vi "test Find Missing Hardware Modules.vi"(8 "error in (no error)":errorcluster, 11 "TestCase in":refnum<class "Routing and Faulting Validation Unit Tests.lvclass">) -> (0 "error out":errorcluster, 3 "TestCase out":refnum<class "Routing and Faulting Validation Unit Tests.lvclass">)   [LabVIEW 2020, in "Routing and Faulting Validation Unit Tests.lvclass"]
uses:
  Routing and Faulting Validation Unit Tests.lvclass
  Routing and Faulting Validation Unit Tests.lvclass/Routing and Faulting Validation Unit Tests.ctl
  <vilib>/addons/_JKI Toolkits/VI Tester/TestCase.llb/TestCase.lvclass
  Routing and Faulting Scripting.lvlib
  C:/Program Files (x86)/National Instruments/LabVIEW 2020/vi.lib/addons/_JKI Toolkits/VI Tester/TestCase.llb/TestCase.lvclass
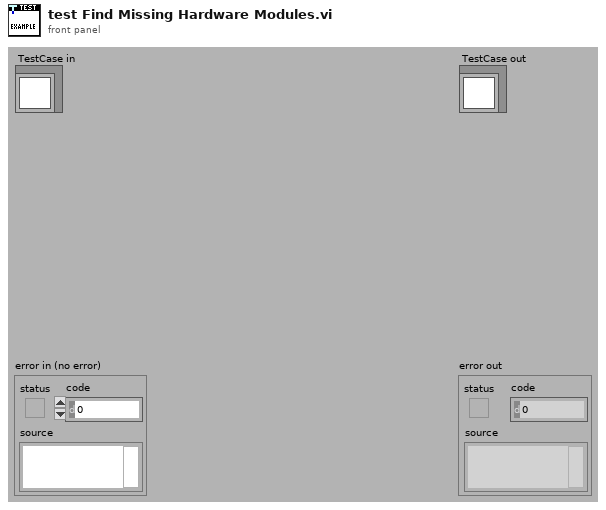
[diagram p1: front panel]
types:
  T1 = typedef "Custom Device API.lvlib/Custom Device Item Ref.ctl" = u64
  T2 = typedef "Routing and Faulting Scripting.lvlib/Validation Information.ctl" = cluster{"Missing Modules":variant, "Module Connection Map":variant, "Unused Modules":variant}
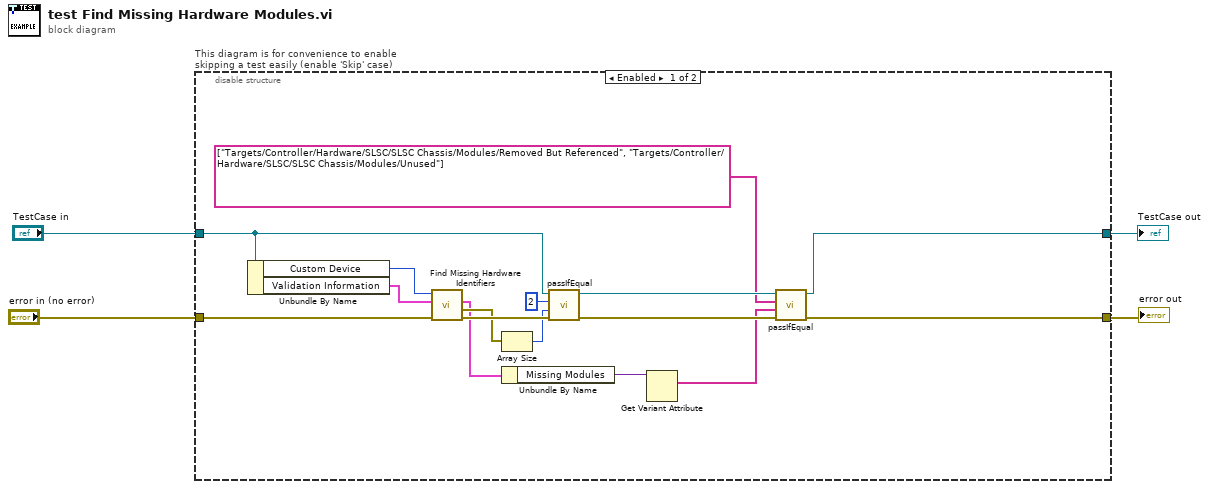
[diagram p0: block diagram]
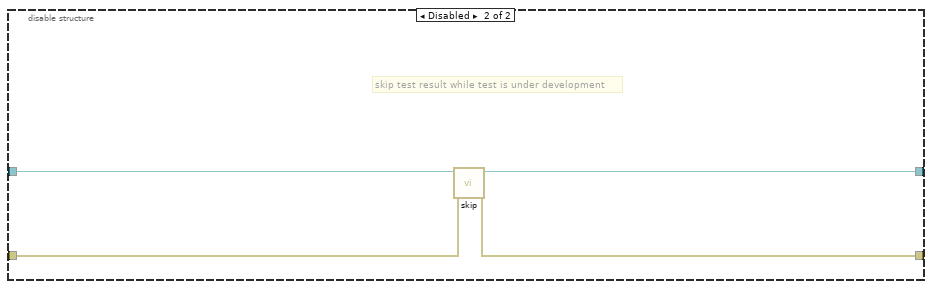
[diagram p2: hidden frame]
diagram:
  n1 = disable-structure "This diagram is for convenience to enable skipping a test easily (enable 'Skip' case)" shown="Enabled" {
    disable-tunnel: "TestCase in" -> [w13 w24]
    disable-tunnel: [w8 w22] -> w1
    disable-tunnel: [w7 w23] -> w3
    disable-tunnel: "error in (no error)" -> [w20 w21]
    frame Enabled {
      n2 = Unbundle By Name(w13) -> ("Custom Device"=w19:T1, "Validation Information"=w18:T2)
      n3 = call "Find Missing Hardware Identifiers.vi"("error in"=w20, "validation information in"=w18, "routing and faulting in"=w19) -> ("error out"=w17:errorcluster, "identifier errors"=w16:errorcluster[], "validation information out"=w12:T2)  [unwired: 5 in, 1 out]
      n4 = Array Size(array=w16) -> (size(s)=w15:i32)
      n5 = Unbundle By Name(w12) -> ("Missing Modules"=w11:variant)
      n6 = call-dynamic "passIfEqual.vi"("error in (no error)"=w17, "y"=w15, "x"=2 ("size(s)"), "TestCase in"=w13) -> ("error out"=w10:errorcluster, "TestCase out"=w9:refnum<class "Routing and Faulting Validation Unit Tests.lvclass">)  [unwired: 6 in]
      n7 = Get Variant Attribute(Variant=w11) -> (names=w5:string[])  [unwired: 3 in, 3 out]
      n8 = call-dynamic "passIfEqual.vi"("error in (no error)"=w10, "y"=w5, "x"=string[] ["Targets/Controller/Hardware/SLSC/SLSC Chassis/Modules/Removed But Referenced", "Targets/Controller/Hardware/SLSC/SLSC Chassis/Modules/Unused"] ("names"), "TestCase in"=w9) -> ("error out"=w7:errorcluster, "TestCase out"=w8:refnum<class "Routing and Faulting Validation Unit Tests.lvclass">)  [unwired: 6 in]
    }
    frame Disabled {
      # "skip test result while test is under development"
      n9 = call <vilib>:"skip.vi"("error in (no error)"=w21, "TestCase in"=w24) -> ("error out"=w23:errorcluster, "TestCase out"=w22:refnum<class "Routing and Faulting Validation Unit Tests.lvclass">)  [unwired: 8 in]
    }
  }
  "error out" <- w3
  "TestCase out" <- w1
